vi "GitTestLabVIEW.vi"() -> ()   [LabVIEW 2020]
panel:
  in  "Hej":dbl
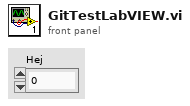
[diagram p1: front panel]
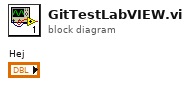
[diagram p0: block diagram]
diagram:
